vi "UIStep Execte UI Resize.vi"(11 "UI Control":T1) -> (3 "UI Control out":T1)   [LabVIEW 2015, in "UIStep.lvclass"]
uses:
  UIStep.lvclass
  <vilib>/Utility/miscctls.llb/LVBoundsTypeDef.ctl
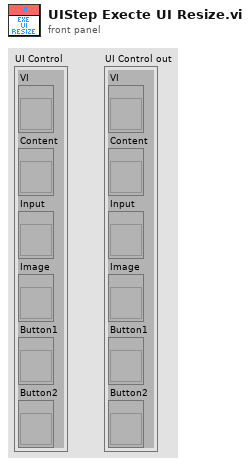
[diagram p1: front panel]
types:
  T1 = cluster{"VI":refnum<vi>, "Content":refnum<vi>, "Input":refnum<vi>, "Image":refnum<vi>, "Button1":refnum<vi>, "Button2":refnum<vi>}
  T2 = typedef "LVBoundsTypeDef.ctl" = cluster{"Width":u32, "Height":u32}
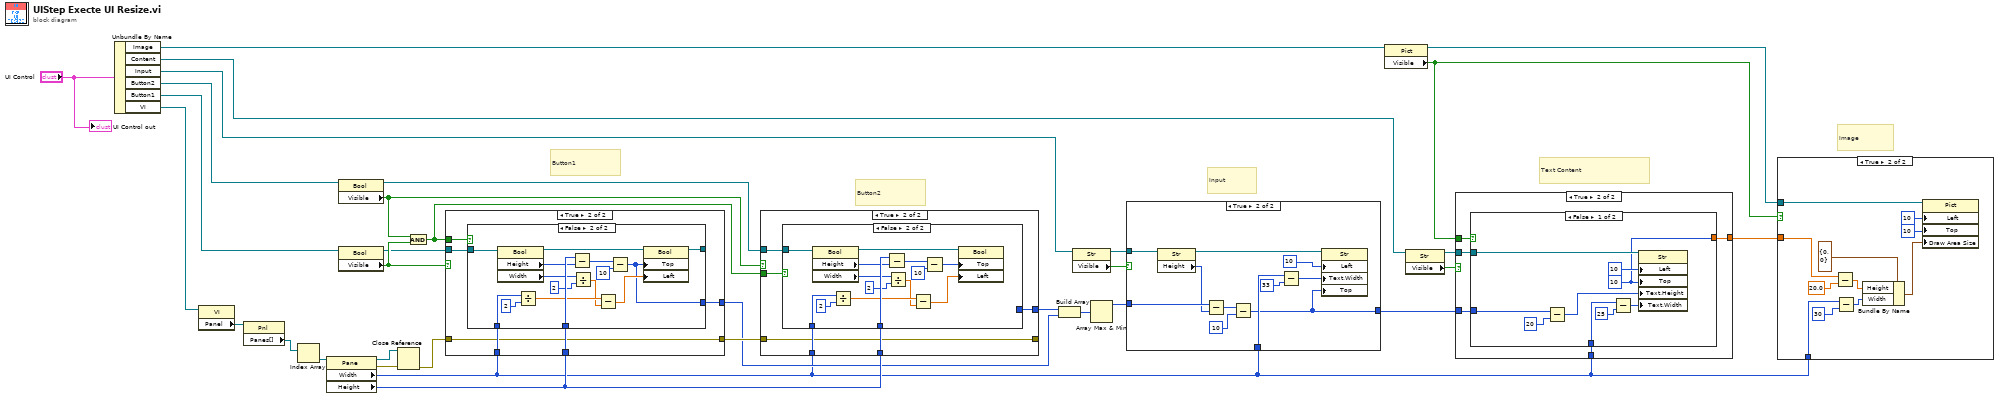
[diagram p0: block diagram]
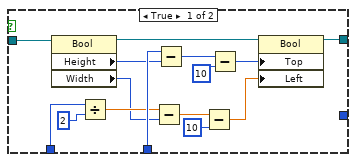
[diagram p3: hidden frame]
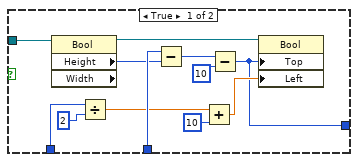
[diagram p5: hidden frame]
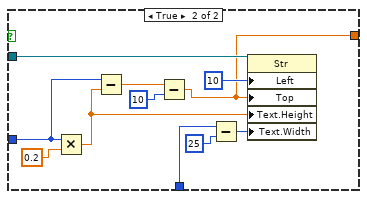
[diagram p9: hidden frame]
diagram:
  # "Image"
  # "Text Content"
  # "Input"
  # "Button2"
  # "Button1"
  n1 = Unbundle By Name("UI Control") -> ("Image"=w7:refnum<vi>, "Content"=w11:refnum<vi>, "Input"=w12:refnum<vi>, "Button2"=w26:refnum<vi>, "Button1"=w27:refnum<vi>, "VI"=w28:refnum<vi>)
  n2 = property class="VI"(reference=w28) -> ("Panel"=w31:refnum<vi>)  [unwired: 1 in, 2 out]
  n3 = property class="Pnl"(reference=w31) -> ("Panes[]"=w30:refnum<vi>[])  [unwired: 1 in, 2 out]
  n4 = Index Array(array=w30) -> (element=w29:refnum<vi>)  [unwired: 1 in]
  n5 = property class="Pane"(reference=w29) -> (reference out=w32:refnum<vi>, error out=w33:errorcluster, "Width"=w3:u32, "Height"=w21:u32)  [unwired: 1 in]
  n6 = property class="Bool"(reference=w26) -> (reference out=w1:refnum<vi>, "Visible"=w23:bool)  [unwired: 1 in, 1 out]
  n7 = property class="Bool"(reference=w27) -> (reference out=w24:refnum<vi>, "Visible"=w25:bool)  [unwired: 1 in, 1 out]
  n8 = Close Reference(reference=w32, error in (no error)=w33) -> (error out=w20:errorcluster)
  n9 = And(x=w23, y=w25) -> (x .and. y?=w22:bool)
  n10 = case shown="True" w25 {
    tunnel: w24 -> [_ w39]
    tunnel: w21 -> [_ w38]
    tunnel: w3 -> [_ w37]
    tunnel: w22 -> [_ w36]
    tunnel: w20 -> [_ w35]
    tunnel: [_ w35] -> w19
    tunnel: [_ w34] -> w17
    frame False {
    }
    frame True {
      n11 = case shown="False" w36 {
        tunnel: w39 -> [w54 w69]
        tunnel: w38 -> [w53 w68]
        tunnel: w37 -> [w47 w63]
        tunnel: [_ w56] -> w34
        tunnel: [w40 w55] -> _
        frame True {
          n12 = property class="Bool"(reference=w54) -> (reference out=w49:refnum<vi>, "Height"=w52:u32, "Width"=w44:u32)  [unwired: 1 in, 1 out]
          n13 = Divide(x=w47, y=2) -> (x/y=w45:dbl)
          n14 = Subtract(x=w45, y=w44) -> (x-y=w43:dbl)
          n15 = Subtract(x=w53, y=w52) -> (x-y=w51:u32)
          n16 = Subtract(x=w43, y=10) -> (x-y=w41:dbl)
          n17 = Subtract(x=w51, y=10) -> (x-y=w48:u32)
          n18 = property class="Bool"(reference=w49, "Top"=w48, "Left"=w41) -> (reference out=w40:refnum<vi>)  [unwired: 1 in, 1 out]
        }
        frame False {
          n19 = property class="Bool"(reference=w69) -> (reference out=w64:refnum<vi>, "Height"=w67:u32, "Width"=w60:u32)  [unwired: 1 in, 1 out]
          n20 = Divide(x=w63, y=2) -> (x/y=w61:dbl)
          n21 = Subtract(x=w68, y=w67) -> (x-y=w66:u32)
          n22 = Divide(x=w60, y=2) -> (x/y=w58:dbl)
          n23 = Subtract(x=w61, y=w58) -> (x-y=w57:dbl)
          n24 = Subtract(x=w66, y=10) -> (x-y=w56:u32)
          n25 = property class="Bool"(reference=w64, "Top"=w56, "Left"=w57) -> (reference out=w55:refnum<vi>)  [unwired: 1 in, 1 out]
        }
      }
    }
  }
  n26 = case shown="True" w23 {
    tunnel: w1 -> [_ w75]
    tunnel: w21 -> [_ w74]
    tunnel: w3 -> [_ w73]
    tunnel: w22 -> [_ w72]
    tunnel: [_ w71] -> _
    tunnel: w19 -> [_ w71]
    tunnel: [_ w70] -> w18
    frame False {
    }
    frame True {
      n27 = case shown="False" w72 {
        tunnel: w75 -> [w87 w101]
        tunnel: w74 -> [w86 w100]
        tunnel: w73 -> [w81 w94]
        tunnel: [w76 _] -> w70
        frame True {
          n28 = property class="Bool" props=["Height", "Width"](reference=w87) -> (reference out=w82:refnum<vi>, "Height"=w85:u32)  [unwired: 1 in, 2 out]
          n29 = Divide(x=w81, y=2) -> (x/y=w77:dbl)
          n30 = Subtract(x=w86, y=w85) -> (x-y=w84:u32)
          n31 = Add(x=w77, y=10) -> (x+y=w78:dbl)
          n32 = Subtract(x=w84, y=10) -> (x-y=w76:u32)
          n33 = property class="Bool"(reference=w82, "Top"=w76, "Left"=w78) -> ()  [unwired: 1 in, 2 out]
        }
        frame False {
          n34 = property class="Bool"(reference=w101) -> (reference out=w96:refnum<vi>, "Height"=w99:u32, "Width"=w91:u32)  [unwired: 1 in, 1 out]
          n35 = Divide(x=w94, y=2) -> (x/y=w92:dbl)
          n36 = Subtract(x=w100, y=w99) -> (x-y=w98:u32)
          n37 = Divide(x=w91, y=2) -> (x/y=w89:dbl)
          n38 = Subtract(x=w92, y=w89) -> (x-y=w88:dbl)
          n39 = Subtract(x=w98, y=10) -> (x-y=w95:u32)
          n40 = property class="Bool"(reference=w96, "Top"=w95, "Left"=w88) -> ()  [unwired: 1 in, 2 out]
        }
      }
    }
  }
  n41 = Build Array(w18, w17) -> (w16:u32[])
  n42 = property class="Str"(reference=w12) -> (reference out=w14:refnum<vi>, "Visible"=w15:bool)  [unwired: 1 in, 1 out]
  n43 = Array Max & Min(array=w16) -> (max value=w13:u32)  [unwired: 3 out]
  n44 = case shown="True" w15 {
    tunnel: w14 -> [_ w109]
    tunnel: w13 -> [w102 w107]
    tunnel: w3 -> [_ w112]
    tunnel: [w102 w103] -> w9
    frame False {
    }
    frame True {
      n45 = property class="Str"(reference=w109) -> (reference out=w108:refnum<vi>, "Height"=w106:u32)  [unwired: 1 in, 1 out]
      n46 = Subtract(x=w107, y=w106) -> (x-y=w105:u32)
      n47 = Subtract(x=w105, y=10 ("Position:Left")) -> (x-y=w103:u32)
      n48 = Subtract(x=w112, y=33) -> (x-y=w110:u32)
      n49 = property class="Str"(reference=w108, "Left"=10 ("Position:Left"), "Text.Width"=w110, "Top"=w103) -> ()  [unwired: 1 in, 2 out]
    }
  }
  n50 = property class="Pict"(reference=w7) -> (reference out=w5:refnum<vi>, "Visible"=w6:bool)  [unwired: 1 in, 1 out]
  n51 = property class="Str"(reference=w11) -> (reference out=w8:refnum<vi>, "Visible"=w10:bool)  [unwired: 1 in, 1 out]
  n52 = case shown="True" w10 {
    tunnel: w9 -> [w114 w116]
    tunnel: w8 -> [_ w119]
    tunnel: w3 -> [_ w118]
    tunnel: w6 -> [_ w117]
    tunnel: [w114 w115] -> w4
    frame False {
    }
    frame True {
      n53 = case shown="False" w117 {
        tunnel: w119 -> [w128 w139]
        tunnel: w118 -> [w126 w137]
        tunnel: w116 -> [w123 w131]
        tunnel: [w120 w132] -> w115
        frame False {
          w120 = 10 ("Position:Top")
          n54 = Subtract(x=w123, y=20) -> (x-y=w121:u32)
          n55 = Subtract(x=w126, y=25) -> (x-y=w124:u32)
          n56 = property class="Str"(reference=w128, "Left"=10 ("Position:Left"), "Top"=w120, "Text.Height"=w121, "Text.Width"=w124) -> ()  [unwired: 1 in, 2 out]
        }
        frame True {
          n57 = Multiply(x=w131, y=0.2) -> (x*y=w129:dbl)
          n58 = Subtract(x=w131, y=w129) -> (x-y=w130:dbl)
          n59 = Subtract(x=w130, y=10 ("Position:Top")) -> (x-y=w132:dbl)
          n60 = Subtract(x=w137, y=25) -> (x-y=w135:u32)
          n61 = property class="Str"(reference=w139, "Left"=10 ("Position:Left"), "Top"=w132, "Text.Height"=w129, "Text.Width"=w135) -> ()  [unwired: 1 in, 2 out]
        }
      }
    }
  }
  n62 = case shown="True" w6 {
    tunnel: w5 -> [_ w150]
    tunnel: w4 -> [_ w145]
    tunnel: w3 -> [_ w147]
    frame False {
    }
    frame True {
      n63 = Subtract(x=w145, y=20.0) -> (x-y=w143:dbl)
      n64 = Subtract(x=w147, y=30) -> (x-y=w141:u32)
      n65 = Bundle By Name(cluster=T2 {"Width"=0, "Height"=0} ("Draw Area Size"), "Height"=w143, "Width"=w141) -> (w140:T2)
      n66 = property class="Pict"(reference=w150, "Left"=10 ("Position:Left"), "Top"=10 ("Position:Top"), "Draw Area Size"=w140) -> ()  [unwired: 1 in, 2 out]
    }
  }
  "UI Control out" <- "UI Control"
